vi "action_controller_a.vi"(0 "Action 1":bool, 1 "Action 2":bool, 2 "Action 3":bool, 3 "Action 4":bool, 4 "First Visible Index":u32) -> (5 "Index":i32, 6 "Action":bool)   [LabVIEW 2017]
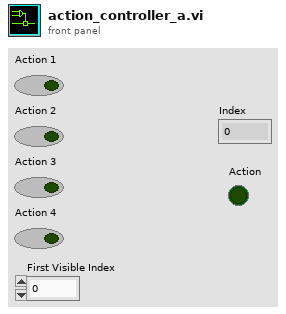
[diagram p1: front panel]
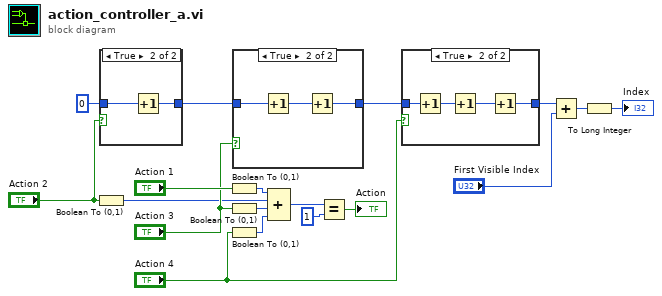
[diagram p0: block diagram]
diagram:
  n1 = Boolean To (0,1)(Boolean="Action 2") -> (0, 1=w10:i16)
  n2 = case shown="True" "Action 2" {
    tunnel: u32 0 -> [w19 w21]
    tunnel: [w19 w20] -> w17
    frame False {
    }
    frame True {
      n3 = Increment(x=w21) -> (x+1=w20:u32)
    }
  }
  n4 = Boolean To (0,1)(Boolean="Action 1") -> (0, 1=w11:i16)
  n5 = Boolean To (0,1)(Boolean="Action 3") -> (0, 1=w9:i16)
  n6 = Boolean To (0,1)(Boolean="Action 4") -> (0, 1=w8:i16)
  n7 = case shown="True" "Action 3" {
    tunnel: w17 -> [w22 w25]
    tunnel: [w22 w23] -> w16
    frame False {
    }
    frame True {
      n8 = Increment(x=w25) -> (x+1=w24:u32)
      n9 = Increment(x=w24) -> (x+1=w23:u32)
    }
  }
  n10 = Compound Arithmetic op=ADD(w11, w10, w9, w8) -> (w7:i16)
  n11 = Equal?(x=w7, y=i16 1) -> (x = y?=→"Action":bool)
  n12 = case shown="True" "Action 4" {
    tunnel: w16 -> [w26 w30]
    tunnel: [w26 w27] -> w1
    frame False {
    }
    frame True {
      n13 = Increment(x=w30) -> (x+1=w29:u32)
      n14 = Increment(x=w29) -> (x+1=w28:u32)
      n15 = Increment(x=w28) -> (x+1=w27:u32)
    }
  }
  n16 = Add(x=w1, y="First Visible Index") -> (x+y=w3:u32)
  n17 = To Long Integer(number=w3) -> (32bit integer=→"Index":i32)
